vi "Read Field - Boolean Array.vi"(7 "field name":string, 8 "error in (no error)":errorcluster, 10 "default":bool[](array[boolean]), 11 "PV Data in":refnum<class "PV Data.lvclass">) -> (0 "error out":errorcluster, 2 "value":bool[](array[boolean]), 3 "PV Data out":refnum<class "PV Data.lvclass">)   [LabVIEW 2020, in "PV Access.lvlib" / "PV Data.lvlib" / "PV Data.lvclass"]
uses:
  PV Data.lvclass
  PV Access.lvlib
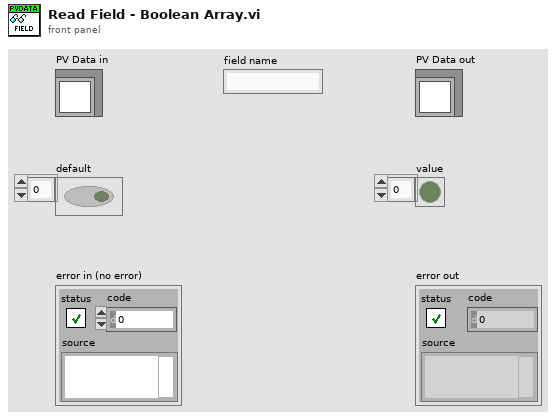
[diagram p1: front panel]
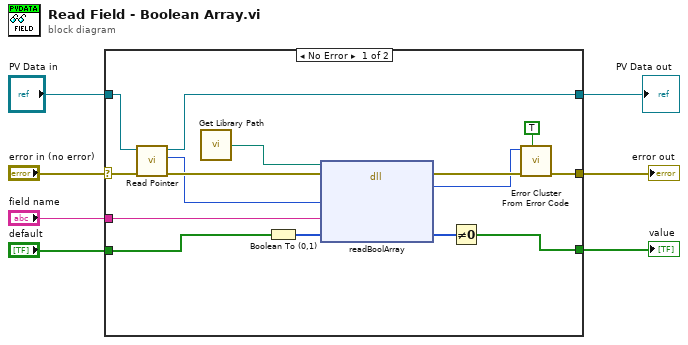
[diagram p0: block diagram]
diagram:
  n1 = case shown="No Error" "error in (no error)" {
    selector: "error in (no error)" -> [w15 w25]
    tunnel: [w16 w25] -> w7
    tunnel: "PV Data in" -> [w13 w24]
    tunnel: [w11 w24] -> w2
    tunnel: "default" -> [w22 w23]
    tunnel: [w21 w23] -> w4
    tunnel: "field name" -> [w10 _]
    frame No Error {
      n2 = call-dynamic "Read Pointer.vi"("error in (no error)"=w15, "Pointer Base in"=w13) -> ("error out"=w14:errorcluster, "Pointer"=w12:i64, "Pointer Base out"=w11:refnum<class "PV Data.lvclass">)  [unwired: 7 in]
      n3 = call "Get Library Path.vi"() -> ("Path"=w20:path)  [unwired: 1 in]
      n4 = Boolean To (0,1)(Boolean=w22) -> (0, 1=w9:i16[])
      n5 = dll-call lib="?" fn="readBoolArray"(path in=w20, error in=w14, "value"=w12, "field_name"=w10, "result"=w9) -> (error out=w18:errorcluster, "err_code"=w17:i32, "result"=w8:i16[])  [unwired: 3 in, 1 out]
      n6 = Not Equal To 0?(x=w8) -> (x != 0?=w21:bool[])
      n7 = call <vilib>:"Error Cluster From Error Code.vi"("show call chain? (False)"=TRUE, "error in (no error)"=w18, "error code (0)"=w17) -> ("error out"=w16:errorcluster)  [unwired: 6 in]
    }
    frame Error {
    }
  }
  "error out" <- w7
  "value" <- w4
  "PV Data out" <- w2
